vi "Initialize.vi"(8 "error in (no error)":errorcluster, 10 "DeviceName":string, 11 "FakePressureController in":refnum<class "TapeMonitor.lvclass">) -> (0 "error out":errorcluster, 1 "new command(s)":string, 2 "DeviceName":string, 3 "FakePressureController out":refnum<class "TapeMonitor.lvclass">)   [LabVIEW 2013, in "TapeMonitor.lvclass"]
uses:
  TapeMonitor.lvclass
  source/Device Driver/BaseDriver/BaseDriver.lvclass
  TapeMonitor.lvclass/TapeMonitor.ctl
panel:
  out "Devicetype\nvariable list":string[][](array[string])
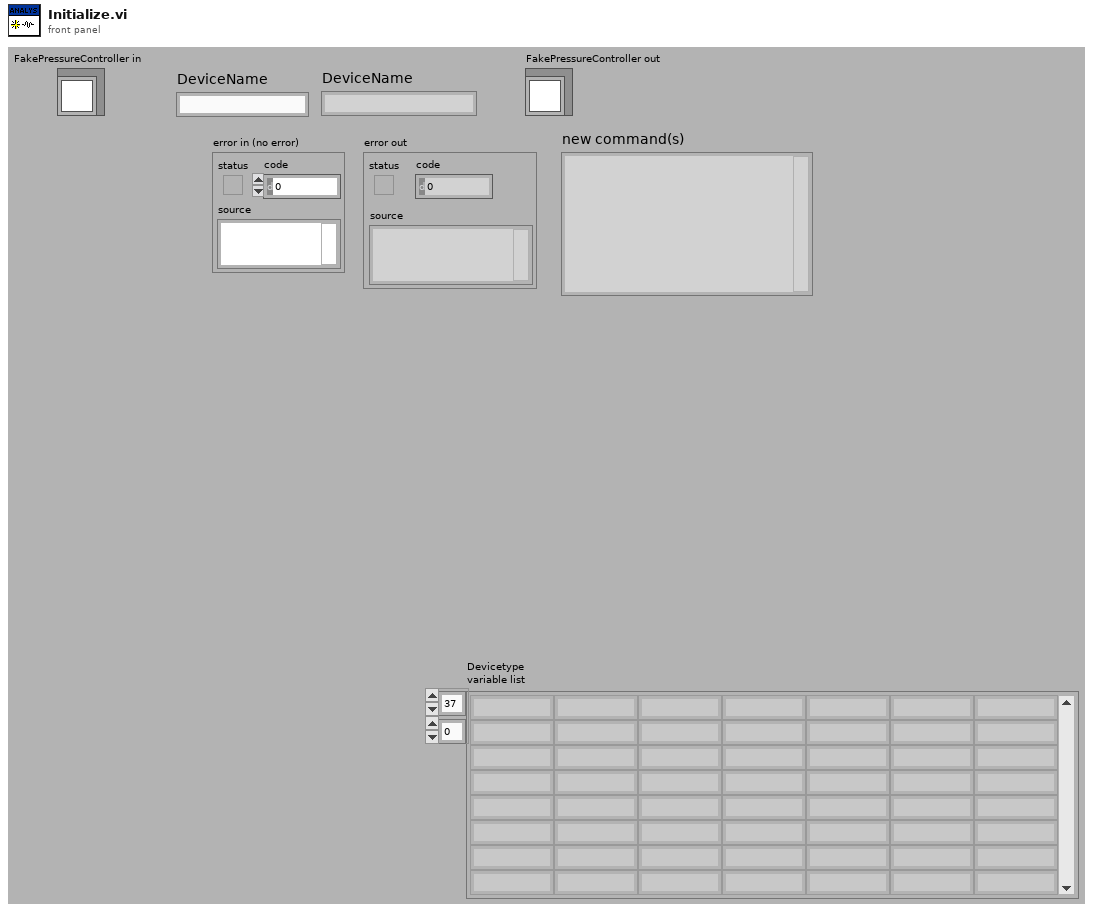
[diagram p1: front panel]
types:
  T1 = typedef "Image Type" = u32
  T2 = typedef "TapeMonitor.lvclass/settings_TypDef.ctl" = cluster{"timeout":T3, "FitnessLimit":T3, "LocalSavingPath":path, "Save":T4, "threshold_low":T3, "threshold_high":T3, "area_min":T3, "area_max":T3}
  T3 = typedef "BaseDriver.lvclass/numericVariable_TypeDef.ctl" = cluster{"Value":dbl, "Min":dbl, "Max":dbl, "StepSize":dbl, "Tolerance":dbl, "ValueActual":dbl}
  T4 = typedef "OnOffTypeDef.ctl" = enum16{"off", "on"}
  T5 = typedef "TapeMonitor.lvclass/analysis_data_typdef.ctl" = cluster{"image":T6}
  T6 = typedef "IMAQ Image.ctl" = refnum<image>
  T7 = typedef "SubscriberCluster_TypDEf.ctl" = cluster{"tcp data event":T8, "Event Registration Refnum":refnum<event-registration>, "data queue":refnum<queue>, "Devices":string[], "Alias":string[], "Variable header":string[], "Devices ALL":string[]}
  T8 = typedef "tcp_new_data_event.ctl" = refnum<user-event>
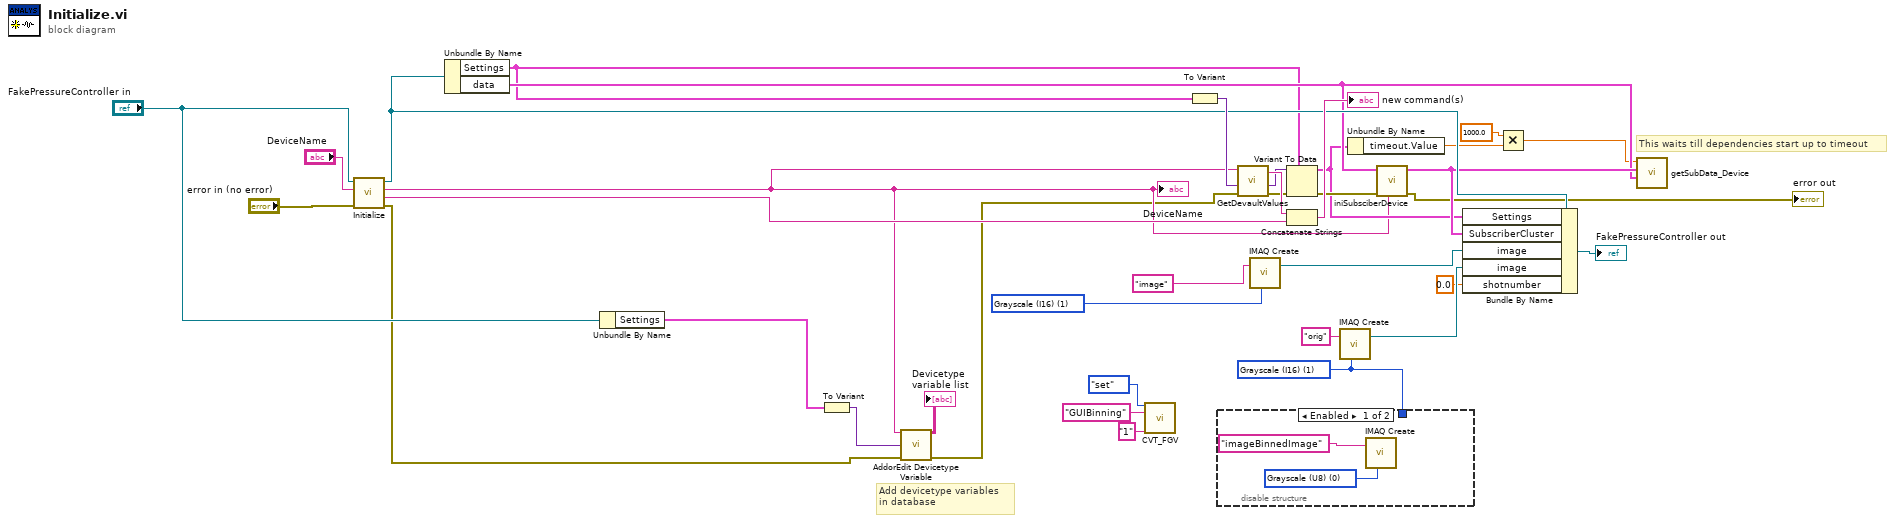
[diagram p0: block diagram]
diagram:
  w16 = T1 1 items=["Grayscale (U8)", "Grayscale (I16)", "Grayscale (SGL)", "Complex (CSG)", "RGB (U32)", "HSL (U32)", "RGB (U64)", "Grayscale (U16)"] ("Image Type")
  w13 = T1 1 items=["Grayscale (U8)", "Grayscale (I16)", "Grayscale (SGL)", "Complex (CSG)", "RGB (U32)", "HSL (U32)", "RGB (U64)", "Grayscale (U16)"] ("Image Type")
  # "Add devicetype variables \nin database"
  # "This waits till dependencies start up to timeout"
  n1 = call-parent "Initialize.vi"("error in (no error)"="error in (no error)", "DeviceName"="DeviceName", "BaseDriver in"="FakePressureController in") -> ("error out"=w3:errorcluster, "new command(s)"=w31:string, "DeviceName"=w6:string, "BaseDriver out"=w27:refnum<class "TapeMonitor.lvclass">)  [unwired: 5 in]
  "DeviceName" <- w6
  n2 = Unbundle By Name(w27) -> ("Settings"=w5:T2, "data"=w24:T5)
  n3 = Unbundle By Name("FakePressureController in") -> ("Settings"=w1:T2)
  n4 = To Variant(anything=w1) -> (Variant=w8:variant)
  n5 = call "AddorEdit Devicetype Variable.vi"("Device Name"=w6, "Settings variant"=w8, "error in"=w3) -> ("Devicetype variable list"=→"Devicetype\nvariable list":string[][], "error out"=w2:errorcluster)  [unwired: 11 in]
  n6 = call "CVT_FGV.vi"("command"=enum16{"set", "get", "reset", "get all"}."set", "variable"="GUIBinning" ("command or variable name"), "value in"="1") -> ()  [unwired: 10 in, 3 out]
  n7 = To Variant(anything=w5) -> (Variant=w32:variant)
  n8 = disable-structure shown="Enabled" {
    disable-tunnel: w13 -> [_ _]
    frame Enabled {
      w37 = T1 0 items=["Grayscale (U8)", "Grayscale (I16)", "Grayscale (SGL)", "Complex (CSG)", "RGB (U32)", "HSL (U32)", "RGB (U64)", "Grayscale (U16)"] ("Image Type")
      n9 = call "IMAQ Create"("Image Name"="imageBinnedImage" ("command or variable name"), "Image Type"=w37) -> ()  [unwired: 3 in, 2 out]
    }
    frame Disabled {
    }
  }
  n10 = call "GetDevaultValues.vi"("error in (no error)"=w2, "variant"=w32, "Device Name"=w6) -> ("error out"=w29:errorcluster, "variant out"=w33:variant, "new command(s)"=w34:string)  [unwired: 6 in]
  n11 = call "IMAQ Create"("Image Name"="image", "Image Type"=w16) -> ("New Image"=w14:T6)  [unwired: 3 in, 1 out]
  n12 = Variant To Data(error in=w29, type=w5, Variant=w33) -> (data=w23:T2, error out=w28:errorcluster)
  n13 = Concatenate Strings(w34, w31) -> (→"new command(s)":string)
  n14 = call "IMAQ Create"("Image Name"="orig", "Image Type"=w13) -> ("New Image"=w17:T6)  [unwired: 3 in, 1 out]
  n15 = Unbundle By Name(w23) -> ("timeout.Value"=w22:dbl)
  n16 = call "iniSubsciberDevice.vi"("DeviceName"=w6, "error in (no error)"=w28, "variant"=w24) -> ("error out"=→"error out":errorcluster, "Subscriber cluster"=w25:T7)  [unwired: 7 in]
  n17 = Bundle By Name(cluster=w27, "Settings"=w23, "SubscriberCluster"=w25, "image"=w14, "image"=w17, "shotnumber"=0.0) -> (→"FakePressureController out":refnum<class "TapeMonitor.lvclass">)
  n18 = Multiply(x=1000.0, y=w22) -> (x*y=w20:dbl)
  n19 = call "getSubData_Device.vi"("variant in"=w24, "SubscriberCluster"=w25, "timeout"=w20) -> ()  [unwired: 7 in, 2 out]
